vi "Set_and_Get.vi"(0 "error in (no error)":errorcluster, 1 "Frequency":dbl) -> (2 "error out":errorcluster, 3 "Amplitude":dbl, 4 "Phase Shift":dbl)   [LabVIEW 2010]
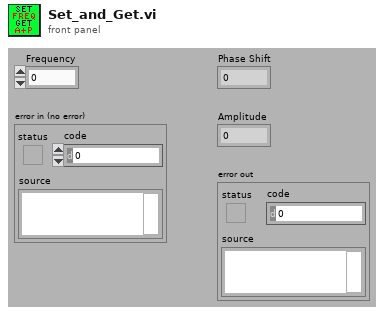
[diagram p1: front panel]
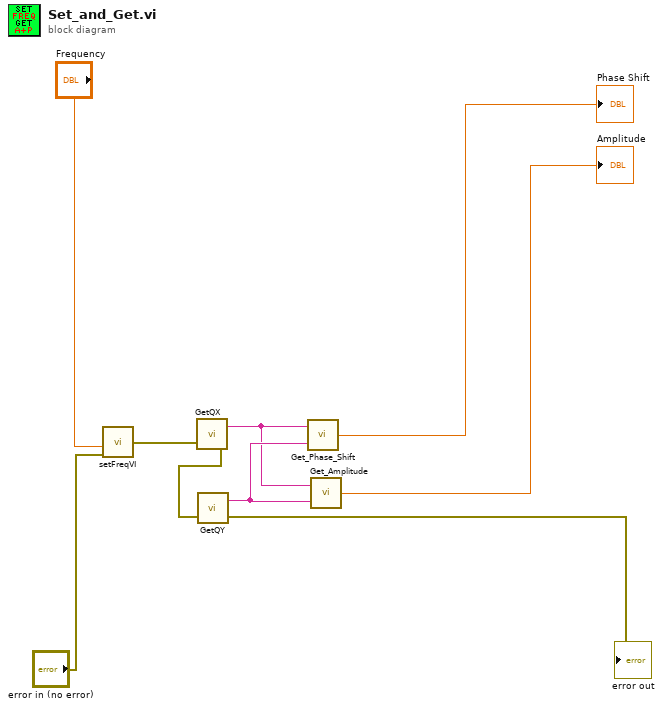
[diagram p0: block diagram]
diagram:
  n1 = call "setFreqVI.vi"("error in"="error in (no error)", "Frequenz in Hz"="Frequency") -> ("error out"=w2:errorcluster)  [unwired: 2 in]
  n2 = call "GetQX.vi"("error in"=w2) -> ("error out"=w3:errorcluster, "data"=w5:string)  [unwired: 1 in]
  n3 = call "GetQY.vi"("error in"=w3) -> ("error out"=→"error out":errorcluster, "data"=w6:string)  [unwired: 1 in]
  n4 = call "Get_Phase_Shift.vi"("Data QY"=w6, "Data QX"=w5) -> ("Numeric"=→"Phase Shift":dbl)
  n5 = call "Get_Amplitude.vi"("Data QY"=w6, "Data QX"=w5) -> ("Numeric"=→"Amplitude":dbl)
